vi "Add_Data_ARCO.vi"(0 "Refnum in":T5, 1 "folder name":string, 2 "historical access":T3={"enable"=FALSE, "queue size (1000)"=1000}, 5 "item 1":T2={"name"="0", "data type"=111, "access level"=3, "description"=""} {"data type" items=["Boolean"=1, "SByte"=2, "Byte"=3, "Int16"=4, "UInt16"=5, "Int32"=6, "UInt32"=7, "Int64"=8, "UInt64"=9, "Float"=10, "Double"=11, "String"=12, "DateTime"=13, "ByteString"=15, "Array of Boolean"=101, "Array of SByte"=102, "Array of Byte"=103, "Array of Int16"=104, "Array of UInt16"=105, "Array of Int32"=106, "Array of UInt32"=107, "Array of Int64"=108, "Array of UInt64"=109, "Array of Float"=110, "Array of Double"=111, "Array of String"=112, "Array of DateTime"=113, "Array of ByteString"=115, "Matrix of Boolean"=201, "Matrix of SByte"=202, "Matrix of Byte"=203, "Matrix of Int16"=204, "Matrix of UInt16"=205, "Matrix of Int32"=206, "Matrix of UInt32"=207, "Matrix of Int64"=208, "Matrix of UInt64"=209, "Matrix of Float"=210, "Matrix of Double"=211, "Matrix of String "=212, "Matrix of DateTime"=213, "Matrix of ByteString"=215]; "access level" items=["read-only"=1, "write-only"=2, "read/write"=3]}, 7 "item 2":T2={"name"="0", "data type"=111, "access level"=3, "description"=""} {"data type" items=["Boolean"=1, "SByte"=2, "Byte"=3, "Int16"=4, "UInt16"=5, "Int32"=6, "UInt32"=7, "Int64"=8, "UInt64"=9, "Float"=10, "Double"=11, "String"=12, "DateTime"=13, "ByteString"=15, "Array of Boolean"=101, "Array of SByte"=102, "Array of Byte"=103, "Array of Int16"=104, "Array of UInt16"=105, "Array of Int32"=106, "Array of UInt32"=107, "Array of Int64"=108, "Array of UInt64"=109, "Array of Float"=110, "Array of Double"=111, "Array of String"=112, "Array of DateTime"=113, "Array of ByteString"=115, "Matrix of Boolean"=201, "Matrix of SByte"=202, "Matrix of Byte"=203, "Matrix of Int16"=204, "Matrix of UInt16"=205, "Matrix of Int32"=206, "Matrix of UInt32"=207, "Matrix of Int64"=208, "Matrix of UInt64"=209, "Matrix of Float"=210, "Matrix of Double"=211, "Matrix of String "=212, "Matrix of DateTime"=213, "Matrix of ByteString"=215]; "access level" items=["read-only"=1, "write-only"=2, "read/write"=3]}, 9 "item 3":T2={"name"="0", "data type"=111, "access level"=3, "description"=""} {"data type" items=["Boolean"=1, "SByte"=2, "Byte"=3, "Int16"=4, "UInt16"=5, "Int32"=6, "UInt32"=7, "Int64"=8, "UInt64"=9, "Float"=10, "Double"=11, "String"=12, "DateTime"=13, "ByteString"=15, "Array of Boolean"=101, "Array of SByte"=102, "Array of Byte"=103, "Array of Int16"=104, "Array of UInt16"=105, "Array of Int32"=106, "Array of UInt32"=107, "Array of Int64"=108, "Array of UInt64"=109, "Array of Float"=110, "Array of Double"=111, "Array of String"=112, "Array of DateTime"=113, "Array of ByteString"=115, "Matrix of Boolean"=201, "Matrix of SByte"=202, "Matrix of Byte"=203, "Matrix of Int16"=204, "Matrix of UInt16"=205, "Matrix of Int32"=206, "Matrix of UInt32"=207, "Matrix of Int64"=208, "Matrix of UInt64"=209, "Matrix of Float"=210, "Matrix of Double"=211, "Matrix of String "=212, "Matrix of DateTime"=213, "Matrix of ByteString"=215]; "access level" items=["read-only"=1, "write-only"=2, "read/write"=3]}, 11 "error in (no error)":errorcluster, 12 "parent folder node ID":T4) -> (4 "Refnum out":T5, 6 "item node ID 1":string, 8 "item node ID 2":string, 10 "item node ID 3":string, 15 "error out":errorcluster)   [LabVIEW 2017]
uses:
  <vilib>/OPCUA/controls/OPC UA Server Refnum.ctl
  <vilib>/OPCUA/controls/NodeId.ctl
  <vilib>/OPCUA/controls/Historical Access.ctl
  <vilib>/OPCUA/controls/Data Type.ctl
  <vilib>/OPCUA/NI OPC UA Server.lvlib
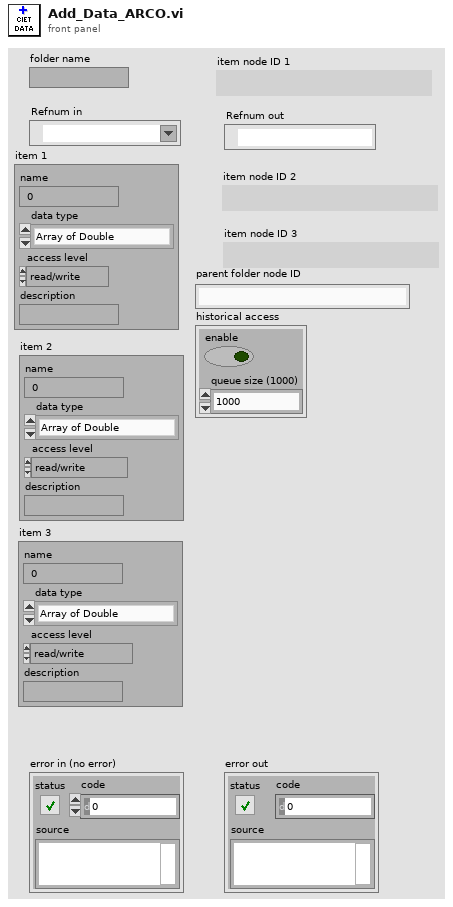
[diagram p1: front panel]
types:
  T1 = typedef "Data Type.ctl" = u16
  T2 = cluster{"name":string, "data type":T1, "access level":u16, "description":string}
  T3 = typedef "Historical Access.ctl" = cluster{"enable":bool, "queue size (1000)":u32}
  T4 = typedef "NodeId.ctl" = string
  T5 = typedef "OPC UA Server Refnum.ctl" = refnum<k21>
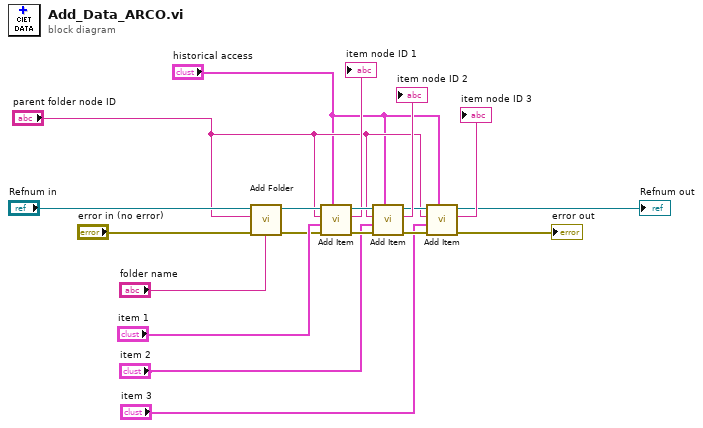
[diagram p0: block diagram]
diagram:
  n1 = call <vilib>:"Add Folder.vi"("error in (no error)"="error in (no error)", "folder name"="folder name", "parent folder node ID"="parent folder node ID", "OPC UA server refnum in"="Refnum in") -> ("error out"=w6:errorcluster, "OPC UA server refnum out"=w5:T5)  [unwired: 4 in, 1 out]
  n2 = call <vilib>:"Add Item.vi"("historical access"="historical access", "error in (no error)"=w6, "item"="item 1", "parent folder node ID"="parent folder node ID", "OPC UA server refnum in"=w5) -> ("error out"=w15:errorcluster, "item node ID"=→"item node ID 1":T4, "OPC UA server refnum out"=w12:T5)  [unwired: 2 in, 1 out]
  n3 = call <vilib>:"Add Item.vi"("historical access"="historical access", "error in (no error)"=w15, "item"="item 2", "parent folder node ID"="parent folder node ID", "OPC UA server refnum in"=w12) -> ("error out"=w16:errorcluster, "item node ID"=→"item node ID 2":T4, "OPC UA server refnum out"=w13:T5)  [unwired: 2 in, 1 out]
  n4 = call <vilib>:"Add Item.vi"("historical access"="historical access", "error in (no error)"=w16, "item"="item 3", "parent folder node ID"="parent folder node ID", "OPC UA server refnum in"=w13) -> ("error out"=→"error out":errorcluster, "item node ID"=→"item node ID 3":T4, "OPC UA server refnum out"=→"Refnum out":T5)  [unwired: 2 in, 1 out]
